vi "filterBallVelocityPeak.vi"(5 "last_balls":T1[](array[typedef]), 6 "ball_id":u32, 7 "dt":dbl, 8 "error in (no error)":errorcluster, 9 "vel_y":dbl, 10 "vel_x":dbl, 11 "Vision in":refnum<class "Vision.lvclass">) -> (0 "error out":errorcluster, 1 "vel_y out":dbl, 2 "vel_x out":dbl, 3 "Vision out":refnum<class "Vision.lvclass">)   [LabVIEW 2020, in "Vision.lvclass"]
uses:
  Vision.lvclass
  Old vision/Controls/SSL Detection Ball.ctl
  <vilib>/Analysis/Matrix/Datatypes/RealMatrix.ctl
  <vilib>/Analysis/Matrix/NI_Matrix.lvlib
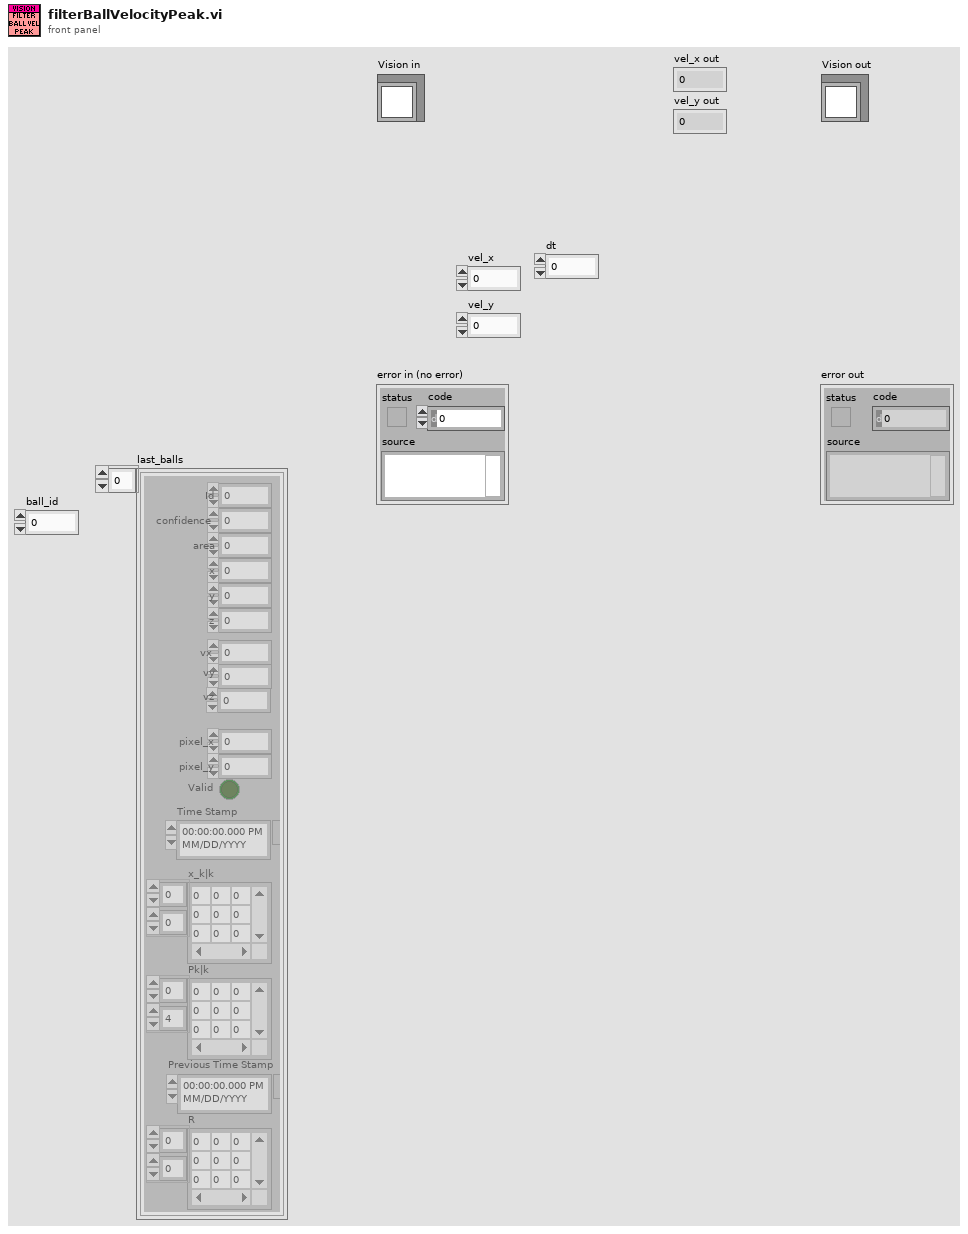
[diagram p1: front panel]
types:
  T1 = typedef "SSL Detection Ball.ctl" = cluster{"x":sgl, "area":u32, "confidence":sgl, "y":sgl, "z":sgl, "pixel_x":sgl, "pixel_y":sgl, "Valid":bool, "Time Stamp":timestamp, "x_k|k":T2, "Pk|k":T2, "Id":u32, "Previous Time Stamp":timestamp, "R":T2, " vx":sgl, "vy":dbl, "vz":dbl}
  T2 = typedef "NI_Matrix.lvlib/RealMatrix.ctl" = dbl[][]
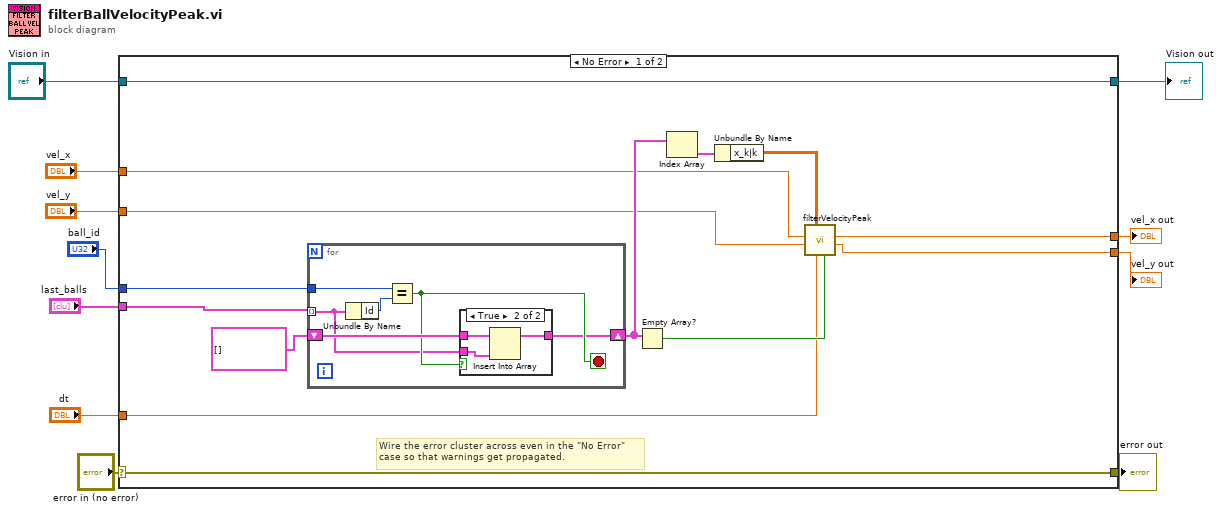
[diagram p0: block diagram]
diagram:
  n1 = case shown="No Error" "error in (no error)" {
    selector: "error in (no error)" -> [w24 w37]
    tunnel: [w24 w37] -> w10
    tunnel: [w25 w36] -> w8
    tunnel: "Vision in" -> [w25 w36]
    tunnel: "ball_id" -> [w22 _]
    tunnel: "last_balls" -> [w21 _]
    tunnel: "vel_x" -> [w16 _]
    tunnel: "dt" -> [w15 _]
    tunnel: "vel_y" -> [w14 _]
    tunnel: [w13 _] -> w2
    tunnel: [w12 _] -> w1
    frame No Error {
      # "Wire the error cluster across even in the \"No Error\"\ncase so that warnings get propagated."
      n2 = for {
        tunnel: w21 -> [w27] mode=indexing
        tunnel: w22 -> [w31]
        shift-right: [w26] -> w20
        shift-left: T1[] [] ("balls") -> [w29]
        stop <- w28 stop-if-true
        n3 = Unbundle By Name(w27) -> ("Id"=w30:u32)
        n4 = Equal?(x=w31, y=w30) -> (x = y?=w28:bool)
        n5 = case shown="True" w28 {
          tunnel: w29 -> [w32 w35]
          tunnel: w27 -> [_ w34]
          tunnel: [w32 w33] -> w26
          frame False {
          }
          frame True {
            n6 = Insert Into Array(array=w35, new element=w34) -> (w33:T1[])  [unwired: 1 in]
          }
        }
      }
      n7 = Empty Array?(array=w20) -> (empty?=w17:bool)
      n8 = Index Array(array=w20) -> (element=w19:T1)  [unwired: 1 in]
      n9 = Unbundle By Name(w19) -> ("x_k|k"=w18:T2)
      n10 = call "filterVelocityPeak.vi"("empty?"=w17, "dt"=w15, "x_k|k"=w18, "vel_y"=w14, "vel_x"=w16) -> ("vel_y out"=w12:dbl, "vel_x out"=w13:dbl)  [unwired: 3 in, 2 out]
    }
    frame Error {
    }
  }
  "error out" <- w10
  "Vision out" <- w8
  "vel_x out" <- w2
  "vel_y out" <- w1
